vi "Temperaturmessung.vi"() -> ()   [LabVIEW 2020]
panel:
  in  "Beiwert":dbl
  in  "Masse":dbl
  out "Signalverlaufsdiagramm":dynamicdata(graph)
  in  "Format-String":string="%f\\t%f\\t%f\\t%f\\t%f\\t\\n"
  in  "Pfad":path=path "C:/Users/Messlabor_Kustos/Desktop/test.xls"
  in  "?":dbl
  in  "Stopp":bool
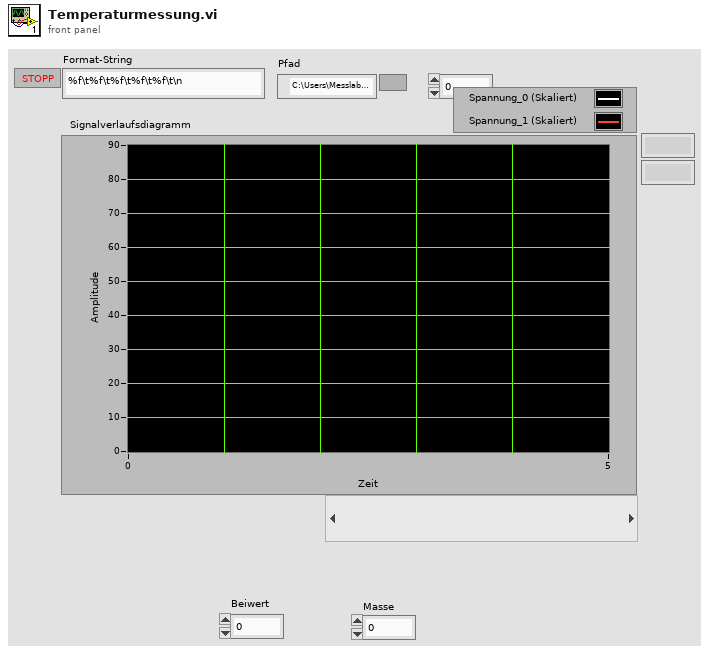
[diagram p1: front panel]
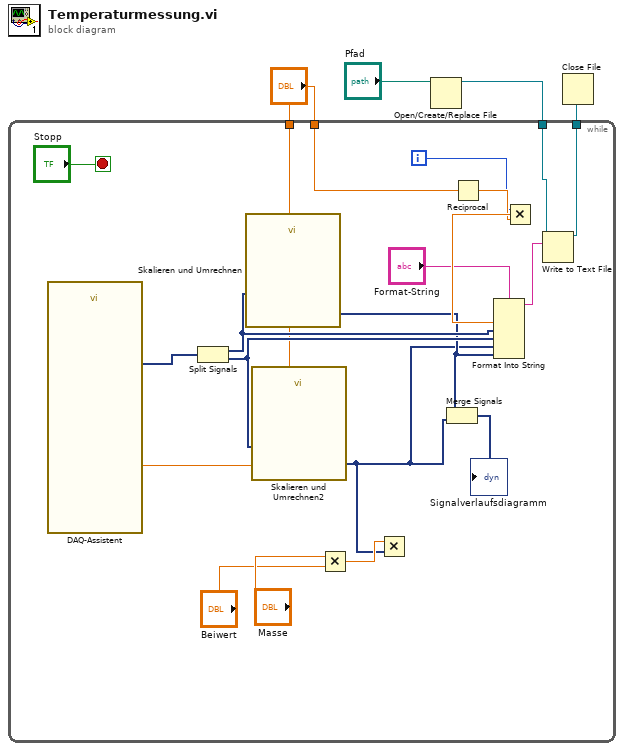
[diagram p0: block diagram]
diagram:
  n1 = Open/Create/Replace File(file path (use dialog)="Pfad") -> (refnum out=w3:refnum<file>)  [unwired: 5 in, 2 out]
  n2 = while {
    tunnel: [w18] -> w4
    tunnel: w3 -> [w17]
    tunnel: "?" -> [w12]
    tunnel: "?" -> [w10]
    i -> [w13]
    stop <- "Stopp" stop-if-true
    n3 = call "DAQ-Assistent"("Rate"=w10) -> ("data"=w11:dynamicdata)  [unwired: 15 in, 3 out]
    n4 = Split Signals(w11) -> (w22:dynamicdata, w21:dynamicdata)  [unwired: 2 in]
    n5 = call "Skalieren und Umrechnen"("Signals"=w22) -> ("Scaled Signals"=w8:dynamicdata)  [unwired: 9 in, 1 out]
    n6 = call "Skalieren und Umrechnen2"("Signals"=w21) -> ("Scaled Signals"=w5:dynamicdata)  [unwired: 9 in, 1 out]
    n7 = Multiply(x="Masse", y="Beiwert") -> (x*y=w6:dbl)
    n8 = Multiply(x=w6, y=w5) -> ()  [unwired: 1 out]
    n9 = Merge Signals(w8, w5) -> (→"Signalverlaufsdiagramm":dynamicdata)
    n10 = Reciprocal(x=w12) -> (1/x=w14:dbl)
    n11 = Multiply(x=w13, y=w14) -> (x*y=w20:dbl)
    n12 = Format Into String(format string="Format-String", w20, w22, w21, w5, w8) -> (resulting string=w19:string)  [unwired: 2 in, 1 out]
    n13 = Write to Text File(file (use dialog)=w17, text=w19) -> (refnum out=w18:refnum<file>)  [unwired: 2 in, 2 out]
  }
  n14 = Close File(refnum=w4) -> ()  [unwired: 1 in, 2 out]
